vi "Page_Version_Write.vi"(6 "ctlReferences":T1, 8 "error in (no error)":errorcluster, 11 "Class in":refnum<class "Installer.lvclass">) -> (0 "error out":errorcluster, 3 "Class out":refnum<class "Installer.lvclass">)   [LabVIEW 2020, in "Installer.lvclass"]
uses:
  <vilib>/AppBuilder/IB_Classes/Installer/Installer.lvclass
  <resource>/Framework/Providers/Builds/Installer/Pages/controls/IB_UI_Page_Version_Info_References.ctl
  <resource>/Framework/Providers/Builds/Installer/CDK_sTypeDef_ProductVersion.ctl
  <vilib>/AppBuilder/IB_Classes/Installer/Installer.lvclass/Installer.ctl
panel:
  # "."
  # "."
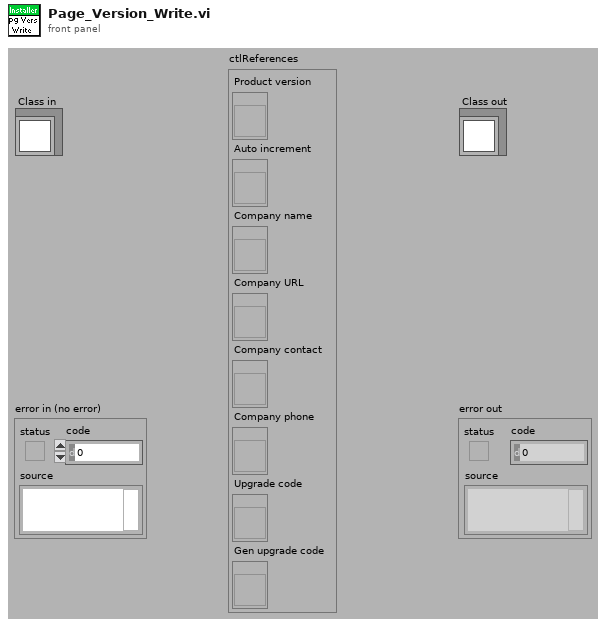
[diagram p1: front panel]
types:
  T1 = typedef "IB_UI_Page_Version_Info_References.ctl" = cluster{"Product version":refnum<vi>, "Auto increment":refnum<vi>, "Company name":refnum<vi>, "Company URL":refnum<vi>, "Company contact":refnum<vi>, "Company phone":refnum<vi>, "Upgrade code":refnum<vi>, "Gen upgrade code":refnum<vi>}
  T2 = typedef "CDK_sTypeDef_ProductVersion.ctl" = cluster{"Major":u8, "Minor":u8, "Update":u16}
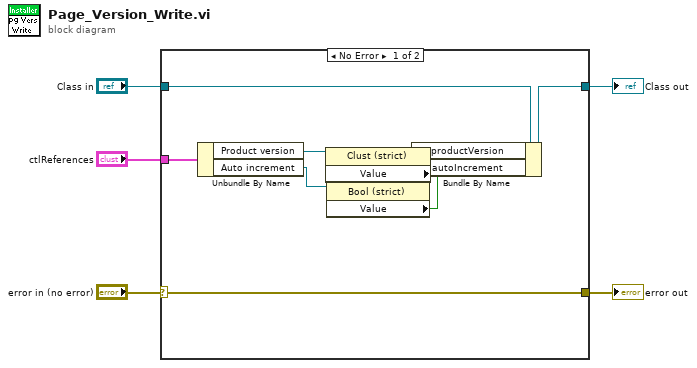
[diagram p0: block diagram]
diagram:
  n1 = case shown="No Error" "error in (no error)" {
    selector: "error in (no error)" -> [w6 w15]
    tunnel: [w6 w15] -> w4
    tunnel: [w11 w14] -> w2
    tunnel: "Class in" -> [w10 w14]
    tunnel: "ctlReferences" -> [w13 _]
    frame No Error {
      n2 = Unbundle By Name(w13) -> ("Product version"=w8:refnum<vi>, "Auto increment"=w12:refnum<vi>)
      n3 = property class="Clust (strict)"(reference=w8) -> ("Value"=w7:T2)  [unwired: 1 in, 2 out]
      n4 = property class="Bool (strict)"(reference=w12) -> ("Value"=w9:bool)  [unwired: 1 in, 2 out]
      n5 = Bundle By Name(cluster=w10, "productVersion"=w7, "autoIncrement"=w9) -> (w11:refnum<class "Installer.lvclass">)
    }
    frame Error {
    }
  }
  "error out" <- w4
  "Class out" <- w2
